vi "DIO open.vi"(8 "error in":errorcluster, 9 "DIO reference":T1) -> (0 "error out":errorcluster, 3 "my FPGA lib.lvlib:DIO.lvclass":refnum<class "DIO.lvclass">)   [LabVIEW 2019, in "my FPGA lib.lvlib" / "DIO.lvclass"]
uses:
  DIO.lvclass
  DIO enum.ctl
  DIO.lvclass/DIO.ctl
  my FPGA lib.lvlib
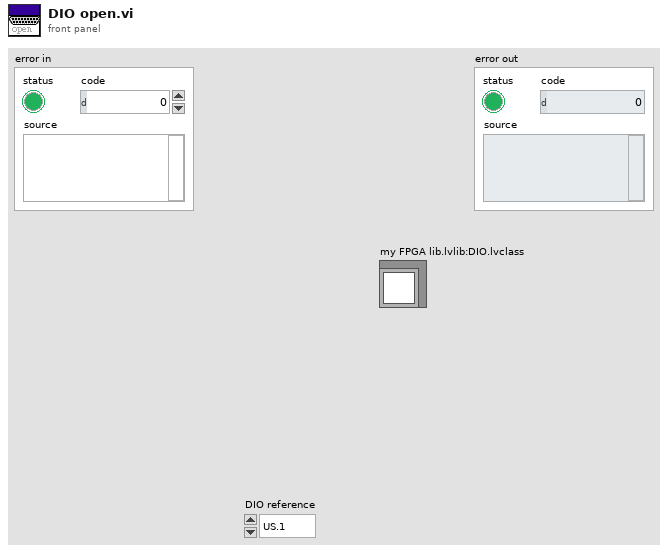
[diagram p1: front panel]
types:
  T1 = typedef "my FPGA lib.lvlib/DIO.lvclass/DIO enum.ctl" = enum16{"US.1", "US.2", "US.3", "US.4", "C.0", "C.1", "C.2", "C.3", "C.4", "C.5", "C.6", "C.7", "B.14", "B.15"}
  T2 = typedef "my FPGA lib.lvlib/DIO.lvclass/port.ctl" = enum16{"US", "C.", "B."}
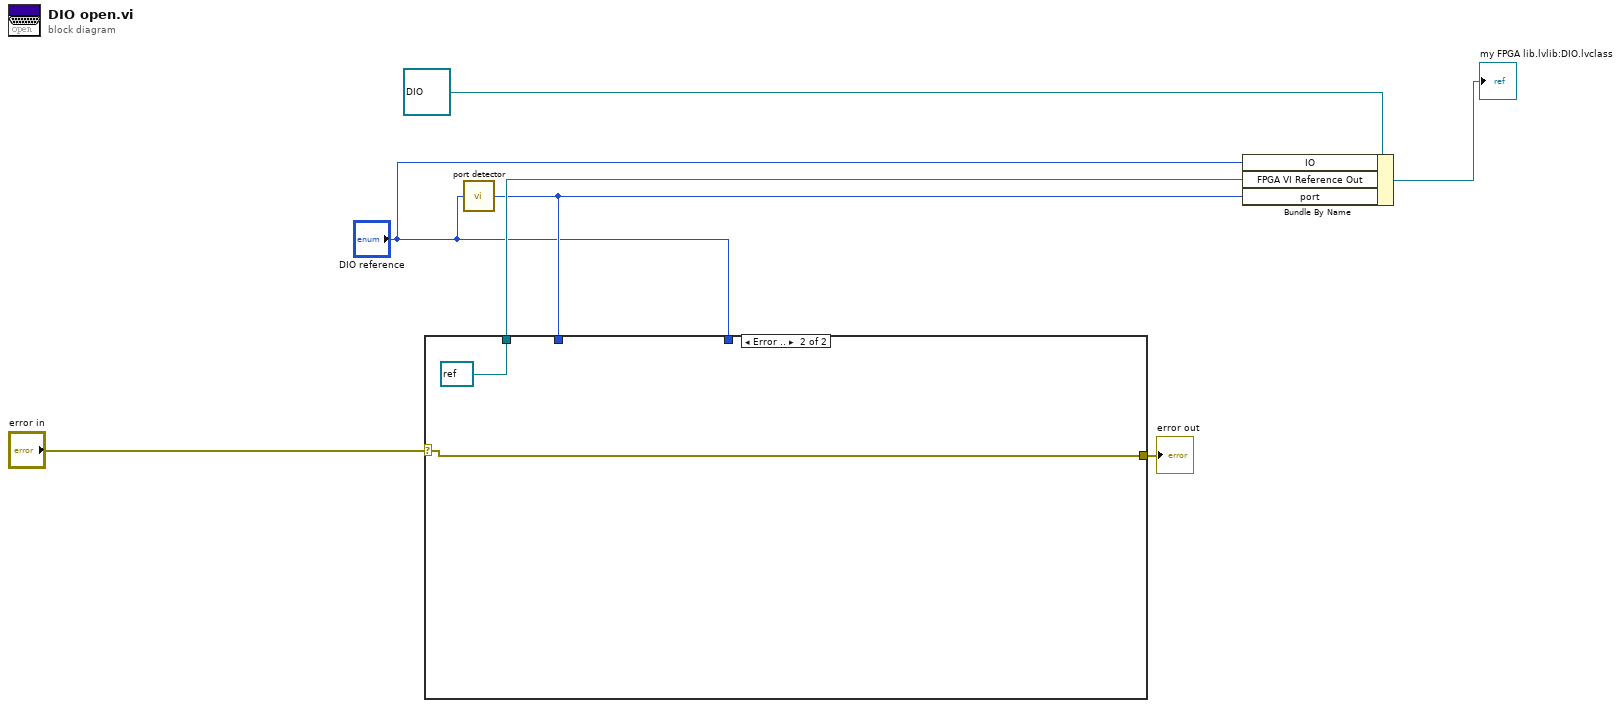
[diagram p0: block diagram]
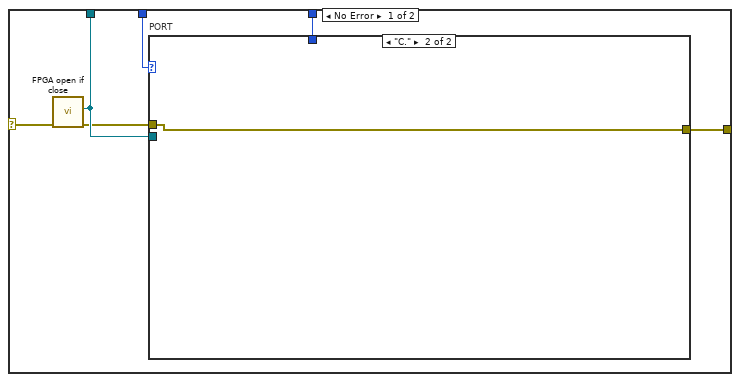
[diagram p2: hidden frame]
diagram:
  n1 = call "port detector.vi"("IO"="DIO reference") -> ("port"=w4:T2)
  n2 = case shown="Error .." "error in" {
    selector: "error in" -> [w13 w18]
    tunnel: [w11 refnum<k20> refnum ("FPGA VI Reference Out")] -> w6
    tunnel: w4 -> [w12 _]
    tunnel: "DIO reference" -> [w9 _]
    tunnel: [w8 w18] -> w1
    frame No Error {
      n3 = call "FPGA open if close.vi"("error in"=w13) -> ("error out"=w10:errorcluster, "FPGA VI Reference Out"=w11:refnum<k20>)  [unwired: 9 in]
      n4 = case "PORT" shown="\"C.\"" w12 {
        tunnel: w11 -> [_ _]
        tunnel: w10 -> [w14 w16]
        tunnel: w9 -> [w15 _]
        tunnel: [w14 w16] -> w8
        frame "US", Default {
          n5 = case shown="\"C.4\"" w15 {
            frame "US.1", Default {
            }
            frame "US.2" {
            }
            frame "US.3" {
            }
            frame "US.4" {
            }
            frame "C.0" {
            }
            frame "C.1" {
            }
            frame "C.2" {
            }
            frame "C.3" {
            }
            frame "C.4" {
            }
          }
        }
        frame "C." {
        }
      }
    }
    frame Error {
    }
  }
  "error out" <- w1
  n6 = Bundle By Name(cluster=refnum<class "DIO.lvclass"> refnum ("my FPGA lib.lvlib:DIO.lvclass"), "IO"="DIO reference", "FPGA VI Reference Out"=w6, "port"=w4) -> (→"my FPGA lib.lvlib:DIO.lvclass":refnum<class "DIO.lvclass">)
